vi "ziUnSubscribe.vi"(3 "error in":errorcluster, 4 "Path (\"/\")":string="/", 5 "Handle in":T1 {"Handle" format="0x%08x"; "Conn" format="0x%08x"}) -> (0 "error out":errorcluster, 2 "Handle out":T1 {"Handle" format="0x%08x"; "Conn" format="0x%08x"})   [LabVIEW 2018, in "Zurich Instruments LabOne.lvlib"]
doc: "This vi is the complement to ziSubscribe.vi. By using wildcards or by using a <b>Path</b> that is not a leaf node but contains sub nodes, more than one node can be unsubscribed with one vi call."
uses:
  Zurich Instruments LabOne.lvlib
  <instrlib>/Zurich Instruments LabOne/Private/ziLV64.framework
  ziTypeHandle.ctl
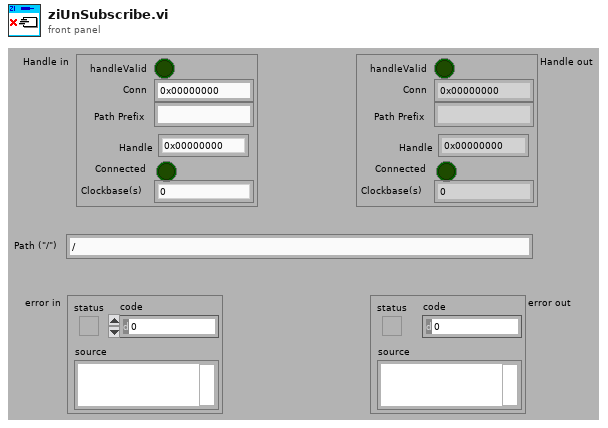
[diagram p1: front panel]
types:
  T1 = typedef "Zurich Instruments LabOne.lvlib/ziTypeHandle.ctl" = cluster{"handleValid":bool, "Conn":u64, "Path Prefix":string, "Handle":u64, "Connected":bool, "Clockbase(s)":dbl}
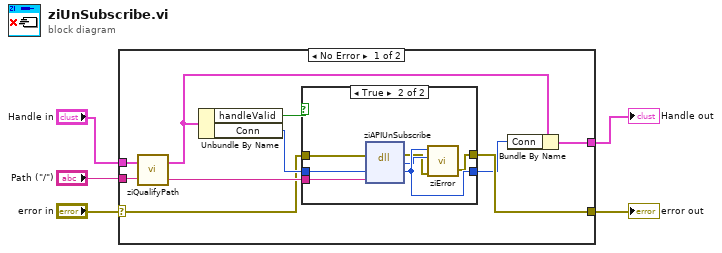
[diagram p0: block diagram]
diagram:
  n1 = case shown="No Error" "error in" {
    selector: "error in" -> [w6 w26]
    tunnel: [w15 w26] -> w5
    tunnel: [w11 w25] -> w4
    tunnel: "Path (\"/\")" -> [w10 _]
    tunnel: "Handle in" -> [w8 w25]
    frame No Error {
      n2 = call "ziQualifyPath.vi"("Path In"=w10, "Handle In"=w8) -> ("Path Out"=w9:string, "Handle Out"=w7:T1)
      n3 = Unbundle By Name(w7) -> ("handleValid"=w14:bool, "Conn"=w13:u64)
      n4 = case shown="True" w14 {
        tunnel: w6 -> [w17 w24]
        tunnel: w13 -> [w16 w23]
        tunnel: [w16 w21] -> w12
        tunnel: [w17 w18] -> w15
        tunnel: w9 -> [_ w22]
        frame False {
        }
        frame True {
          n5 = dll-call lib="Applications/National Instruments/LabVIEW 2019 64-bit/instr.lib/Zurich Instruments LabOne/Private/ziLV*.*" fn="ziAPIUnSubscribe"(error in=w24, "Conn"=w23, "Path"=w22) -> (error out=w19:errorcluster, "return type"=w20:u32, "Conn"=w21:u64)  [unwired: 3 in, 1 out]
          n6 = call "ziError.vi"("Conn"=w21, "ziErrorCode"=w20, "Error In"=w19) -> ("Error Out"=w18:errorcluster)  [unwired: 2 in, 1 out]
        }
      }
      n7 = Bundle By Name(cluster=w7, "Conn"=w12) -> (w11:T1)
    }
    frame Error {
    }
  }
  "error out" <- w5
  "Handle out" <- w4
